vi "List settings enum.vi"(7 "setting enum reference":refnum<vi>, 8 "error in (no error)":errorcluster, 11 "ServiceManager in":refnum<class "ServiceManager.lvclass">) -> (0 "error out":errorcluster, 3 "ServiceManager out":refnum<class "ServiceManager.lvclass">)   [LabVIEW 2012, in "ServiceManager.lvclass"]
uses:
  ServiceManager.lvclass
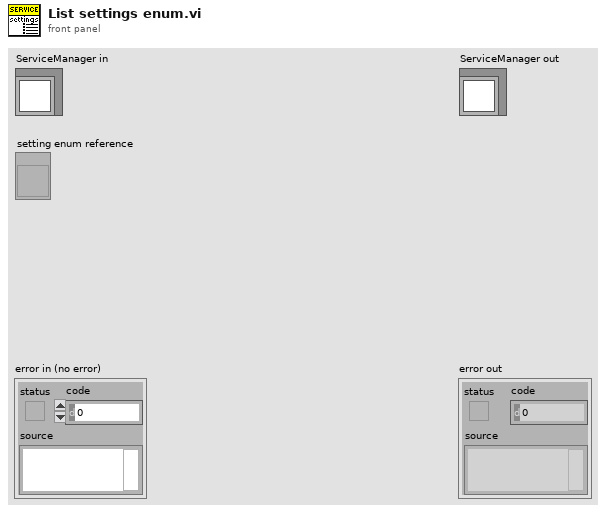
[diagram p1: front panel]
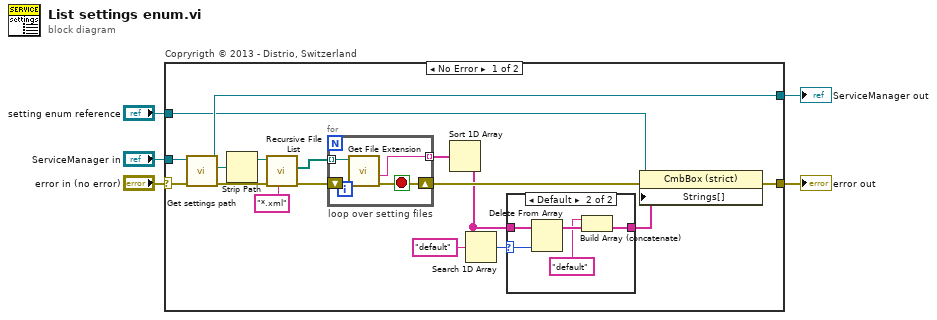
[diagram p0: block diagram]
diagram:
  n1 = case "Copryrigth © 2013 - Distrio, Switzerland" shown="No Error" "error in (no error)" {
    selector: "error in (no error)" -> [w22 w34]
    tunnel: [w13 w34] -> w4
    tunnel: [w20 w33] -> w2
    tunnel: "ServiceManager in" -> [w21 w33]
    tunnel: "setting enum reference" -> [w15 _]
    frame No Error {
      n2 = call-dynamic "Get settings path.vi"("error in (no error)"=w22, "Murmex in"=w21) -> ("error out"=w18:errorcluster, "settings path"=w6:path, "Murmex out"=w20:refnum<class "ServiceManager.lvclass">)  [unwired: 7 in]
      n3 = Strip Path(path=w6) -> (stripped path=w7:path)  [unwired: 1 out]
      n4 = call <vilib>:"Recursive File List.vi"("pattern"="*.xml", "error in (no error)"=w18, "Folder Path"=w7) -> ("error out"=w16:errorcluster, "All Files in Dir"=w17:path[])  [unwired: 4 in, 3 out]
      n5 = for "loop over setting files" {
        tunnel: w17 -> [w32] mode=indexing
        tunnel: [w30] -> w12 mode=indexing
        shift-right: [w29] -> w14
        shift-left: w16 -> [w31]
        stop <- w29 stop-if-true
        n6 = call <vilib>:"Get File Extension.vi"("error in (no error)"=w31, "file"=w32) -> ("error out"=w29:errorcluster, "filename without extension"=w30:string)  [unwired: 6 in, 2 out]
      }
      n7 = Sort 1D Array(array=w12) -> (sorted array=w10:string[])
      n8 = Search 1D Array(1D array=w10, element="default") -> (index of element=w9:i32)  [unwired: 1 in]
      n9 = case shown="Default" w9 {
        selector: w9 -> [_ w27]
        tunnel: w10 -> [w23 w28]
        tunnel: [w23 w24] -> w8
        frame -1 {
        }
        frame Default {
          n10 = Delete From Array(array=w28, index=w27) -> (array with subset deleted=w26:string[])  [unwired: 1 in, 1 out]
          n11 = Build Array (concatenate)("default" ("element"), w26) -> (w24:string[])
        }
      }
      n12 = property class="CmbBox (strict)"(reference=w15, error in=w14, "Strings[]"=w8) -> (error out=w13:errorcluster)  [unwired: 1 out]
    }
    frame Error {
    }
  }
  "error out" <- w4
  "ServiceManager out" <- w2
